vi "信号显示.vi"() -> ()   [LabVIEW 2014]
panel:
  in  "旋钮":dbl(knob) scale=0.0..10.0
  in  "转盘":dbl(knob) scale=0.0..10.0
  in  "选项卡控件":enum32{"选项卡 1", "选项卡 2"}(tab)
  in  "信号类型":enum16{"Sine Wave"}(ring)
  in  "频率":dbl(knob) scale=0.0..50.0
  in  "幅值":dbl(knob) scale=0.0..10.0
  in  "相位":dbl(knob) scale=0.0..50.0
  in  "开启/关闭噪声":bool
  in  "噪声幅值":dbl(knob) scale=0.0..50.0
  in  "噪声选择":enum16{"均匀白噪声"}(ring)
  in  "均值(泊松)":dbl
  in  "高斯白噪声偏差":dbl
  in  "数值 3":dbl
  in  "确定按钮":bool
  in  "主页按钮":bool
  in  "停止按钮":bool
  out "输入信号":dbl[](graph)
  out "幅值":dbl[](graph)
  out "实部":dbl[](graph)
  out "相位":dbl[](graph)
  out "虚部":dbl[](graph)
  out "周期信号":bool
  out "非周期信号":bool
  out "运行":bool
  out "噪声":bool
  in  "字符串":string
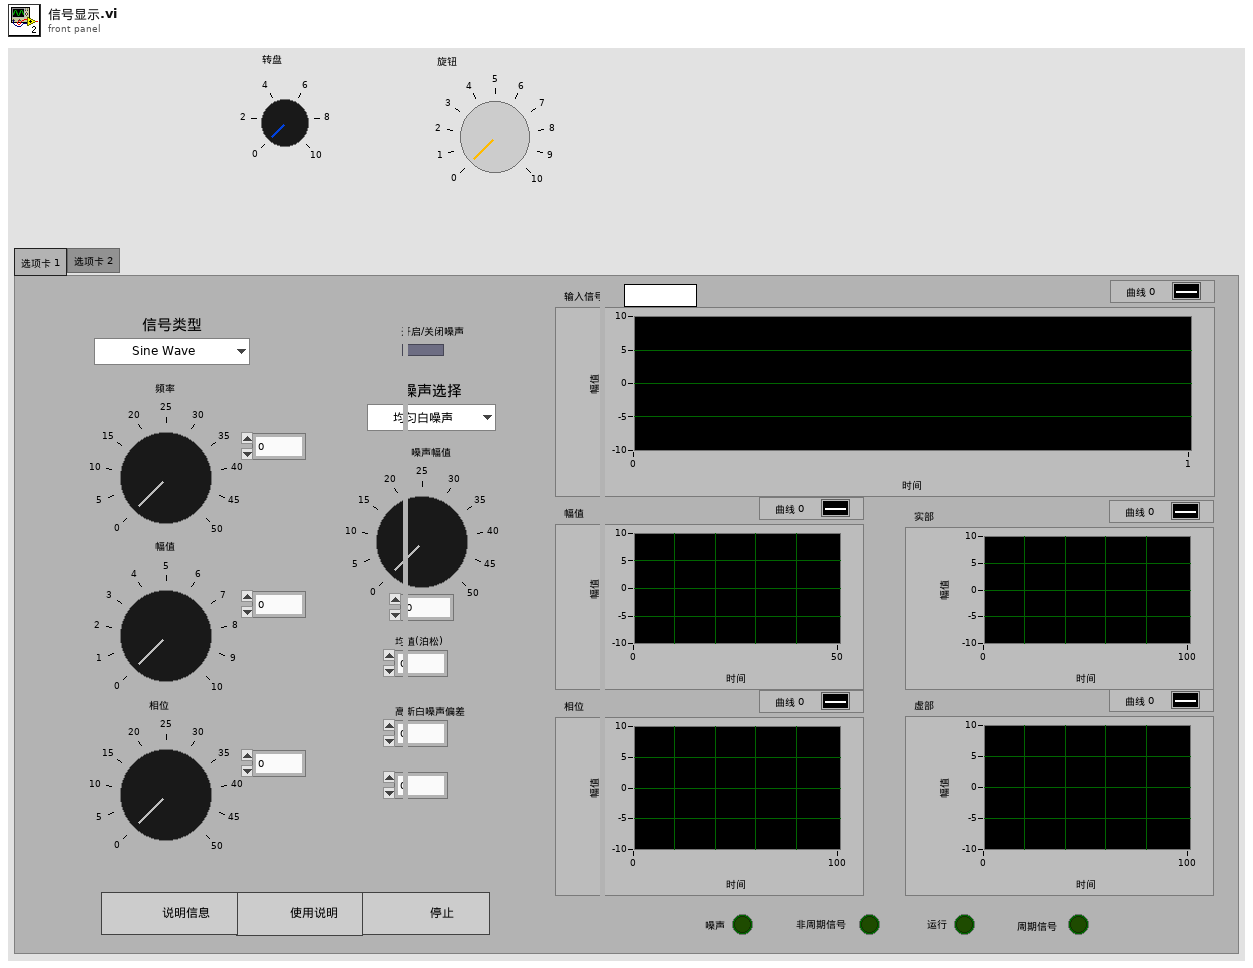
[diagram p1: front panel]
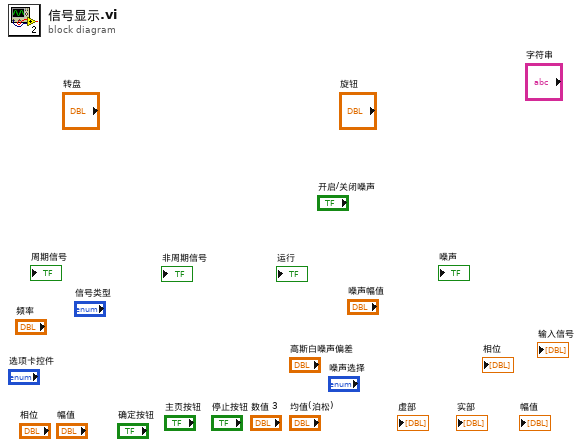
[diagram p0: block diagram]
diagram:
